vi "Create.vi"(8 "error in (no error)":errorcluster, 11 "TopLevel in":refnum<class "IO.lvclass">) -> (0 "error out":errorcluster, 3 "TopLevel out":refnum<class "IO.lvclass">)   [LabVIEW 2022 SP3, in "IO.lvclass"]
uses:
  IO.lvclass
  IO.lvclass/IO.ctl
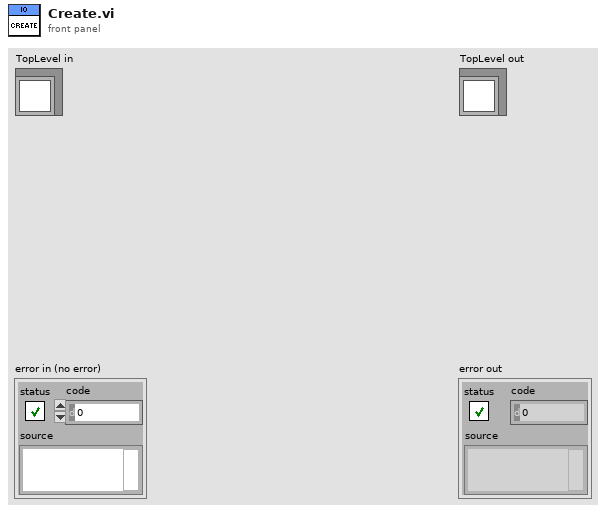
[diagram p1: front panel]
types:
  T1 = typedef "IO.lvclass/Private Data.ctl" = cluster{"UserEvents":T2, "All Dependencies":cluster{"Class References":refnum<class>[], "Class Names":string[]}, "Status":T3}
  T2 = typedef "IO.lvclass/UserEvents.ctl" = cluster{"API Incoming Event":refnum<user-event>, "API Executed Event":refnum<user-event>, "API Return Event":refnum<user-event>, "Status Changed Event":refnum<user-event>}
  T3 = typedef "IO.lvclass/Status Cluster.ctl" = cluster{"Device Data":variant, "Ordered ICP1-DO Channels":T4[], "Ordered ICP2-DI Channels":T5[], "Ordered ICP2-DO Channels":T6[], "Ordered ICP1-AI Channels":T7[], "Ordered ICP1-AO Channels":T8[], "Ordered ICP2-AO Channels":T9[]}
  T4 = typedef "IO.lvclass/ICP1-D0 Channel Names.ctl" = enum16{"None", "Meniscus Pressure Reg PWR - R1", "Meniscus Pressure Reg PWR - R2", "Meniscus Pressure Reg PWR - R3", "Meniscus Pressure Reg PWR - R4", "Meniscus Pressure Reg PWR - R5", "Meniscus Pressure Reg PWR - R6", "Clear Stage Alarm", "Servo ON", "Purge Valve Open - R1", "Purge Valve Open - R2", "Purge Valve Open - R3", "Purge Valve Open - R4", "Purge Valve Open - R5", "Purge Valve Open - R6"}
  T5 = typedef "IO.lvclass/ICP2-DI Channel Names.ctl" = enum16{"None", "SW - Ink Valve - R1", "SW - Ink Valve - R2", "SW - Ink Valve - R3", "SW - Ink Valve - R4", "SW - Ink Valve - R5", "SW - Ink Valve - R6", "SW - COVER INPUT SIDE", "SW - COVER OUTPUT SIDE", "SW - Purge - R1", "SW - Purge - R2", "SW - Purge - R3", "SW - Purge - R4", "SW - Purge - R5", "SW - Purge - R6"}
  T6 = typedef "IO.lvclass/ICP2-DO Channel Names.ctl" = enum16{"None", "Meniscus Valve Open - R1", "Meniscus Valve Open - R2", "Meniscus Valve Open - R3", "Meniscus Valve Open - R4", "Meniscus Valve Open - R5", "Meniscus Valve Open - R6", "Ink Flow Valve Open - R1", "Ink Flow Valve Open - R2", "Ink Flow Valve Open - R3", "Ink Flow Valve Open - R4", "Ink Flow Valve Open - R5", "Ink Flow Valve Open - R6", "SW_LED - Ink Valve - R1", "SW_LED - Ink Valve - R2", "SW_LED - Ink Valve - R3", "Recirc Pump On - R1", "Recirc Pump On - R2", "Recirc Pump On - R3", "Recirc Pump On - R4", "Recirc Pump On - R5", "Recirc Pump On - R6", "SW_LED - Ink Valve - R4", "SW_LED - Ink Valve - R5", "SW_LED - Ink Valve - R6"}
  T7 = typedef "IO.lvclass/ICP1-AI Channel Names.ctl" = enum16{"None", "Meniscus Pressure Read - R1", "Meniscus Pressure Read - R2", "Meniscus Pressure Read - R3", "Meniscus Pressure Read - R4", "Meniscus Pressure Read - R5", "Meniscus Pressure Read - R6", "Meniscus Pressure Set - R1", "Meniscus Pressure Set - R2", "Meniscus Pressure Set - R3", "Meniscus Pressure Set - R4", "Meniscus Pressure Set - R5", "Meniscus Pressure Set - R6"}
  T8 = typedef "IO.lvclass/ICP1-AO Channel Names.ctl" = enum16{"None", "Meniscus Pressure Set - R1", "Meniscus Pressure Set - R2", "Meniscus Pressure Set - R3", "Meniscus Pressure Set - R4", "Meniscus Pressure Set - R5", "Meniscus Pressure Set - R6", "Meniscus Vac Pump Speed"}
  T9 = typedef "IO.lvclass/ICP2-AO Channel Names.ctl" = enum16{"None", "Recirc Pump Flow Set - R1", "Recirc Pump Flow Set - R2", "Recirc Pump Flow Set - R3", "Recirc Pump Flow Set - R4", "Recirc Pump Flow Set - R5", "Recirc Pump Flow Set - R6"}
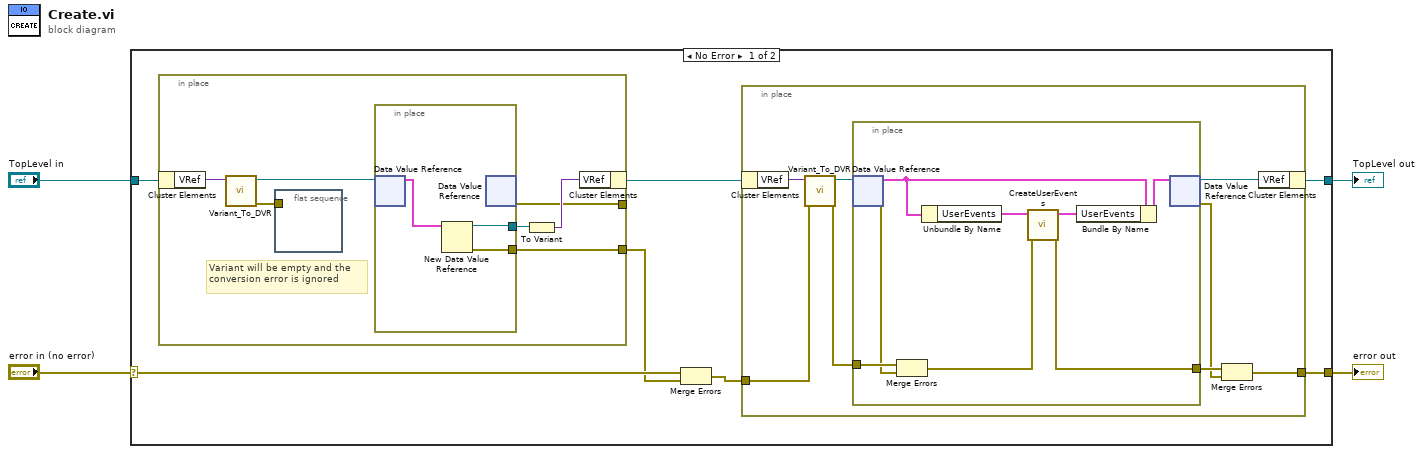
[diagram p0: block diagram]
diagram:
  n1 = case shown="No Error" "error in (no error)" {
    selector: "error in (no error)" -> [w11 w39]
    tunnel: [w5 w39] -> w3
    tunnel: [w7 w38] -> w1
    tunnel: "TopLevel in" -> [w10 w38]
    frame No Error {
      n2 = in-place {
        in-place-border: [w29] -> _
        in-place-border: [w28] -> w9
        # "Variant will be empty and the conversion error is ignored"
        n3 = in-place-cluster #1(w10) -> ("VRef"=w34:variant)
        n4 = call "Variant_To_DVR.vi"("Variant"=w34) -> ("error out"=w33:errorcluster, "DVR"=w32:refnum<data-value>)  [unwired: 9 in]
        n5 = flat-sequence {
          tunnel: w33 -> [_]
          frame #0 {
          }
        }
        n6 = in-place {
          in-place-border: [w36] -> w31
          in-place-border: [w35] -> w28
          n7 = in-place-dvr #2(w32) -> (w37:T1)  [unwired: 1 out]
          n8 = New Data Value Reference(data value=w37) -> (data value reference=w36:refnum<data-value>, error out=w35:errorcluster)  [unwired: 1 in]
          n9 = in-place-dvr #2() -> (w29:errorcluster)  [unwired: 1 in, 1 out]
        }
        n10 = To Variant(anything=w31) -> (Variant=w30:variant)
        n11 = in-place-cluster #1("VRef"=w30) -> (w8:refnum<class "IO.lvclass">)
      }
      n12 = Merge Errors(w11, w9) -> (w6:errorcluster)
      n13 = in-place {
        in-place-border: w6 -> [w17]
        in-place-border: [w13] -> w5
        n14 = in-place-cluster #3(w8) -> ("VRef"=w19:variant)
        n15 = call "Variant_To_DVR.vi"("error in (no error)"=w17, "Variant"=w19) -> ("error out"=w16:errorcluster, "DVR"=w18:refnum<data-value>)  [unwired: 8 in]
        n16 = in-place {
          in-place-border: w16 -> [w23]
          in-place-border: [w20] -> w15
          n17 = in-place-dvr #4(w18) -> (w26:T1, w21:errorcluster)
          n18 = Merge Errors(w23, w21) -> (w22:errorcluster)
          n19 = Unbundle By Name(w26) -> ("UserEvents"=w27:T2)
          n20 = call "CreateUserEvents.vi"("error in (no error)"=w22, "UserEvents"=w27) -> ("error out"=w20:errorcluster, "UserEvents out"=w25:T2)  [unwired: 8 in]
          n21 = Bundle By Name(cluster=w26, "UserEvents"=w25) -> (w24:T1)
          n22 = in-place-dvr #4(w24) -> (w12:refnum<data-value>, w14:errorcluster)
        }
        n23 = Merge Errors(w15, w14) -> (w13:errorcluster)
        n24 = in-place-cluster #3("VRef"=w12) -> (w7:refnum<class "IO.lvclass">)
      }
    }
    frame Error {
    }
  }
  "error out" <- w3
  "TopLevel out" <- w1
